vi "rsscope_core_global.vi"() -> ()   [LabVIEW 2014] (continued)
"Access"=2, "Range Table"="", "Read Callback"="rsscope_FormatSearchNameString_ReadCallback.vi", "Write Callback"="rsscope_FormatSearchNameString_WriteCallback.vi", "Supported Models"="", "Instrument Options"="K44", "Flags"=0, "Help"="Specifies the CRC bit pattern, or sets the start value of a pattern range.\n\nAvailable Repeated Capabilities:\nNone\n\nRemote-control command(s):\nSEARch:TRIGger:MPHY:CRC:MIN"}, {"Level"=4, "Class Only"=FALSE, "Identifier"="RSSCOPE_ATTR_SEARCH_MPHY_CRC_MAX", "Descriptive Name"="Search MPHY CRC Max", "Data Type"=2, "Command"="SEAR:TRIG:MPHY:CRC:MAX", "Access"=2, "Range Table"="", "Read Callback"="rsscope_FormatSearchNameString_ReadCallback.vi", "Write Callback"="rsscope_FormatSearchNameString_WriteCallback.vi", "Supported Models"="", "Instrument Options"="K44", "Flags"=0, "Help"="Sets the end value of the CRC range if SEARch:TRIGger:MPHY:CRC:CONDition is set to In Range or Out Of Range.\n\nAvailable Repeated Capabilities:\nNone\n\nRemote-control command(s):\nSEARch:TRIGger:MPHY:CRC:MAX"}, {"Level"=4, "Class Only"=FALSE, "Identifier"="RSSCOPE_ATTR_SEARCH_MPHY_CREQ_PATTERN", "Descriptive Name"="Search MPHY CREQ Pattern", "Data Type"=0, "Command"="SEAR:TRIG:MPHY:CREQ", "Access"=2, "Range Table"="RsScope_rngMPHYREQPattern", "Read Callback"="rsscope_FormatSearchNameInt32_ReadCallback.vi", "Write Callback"="rsscope_FormatSearchNameInt32_WriteCallback.vi", "Supported Models"="", "Instrument Options"="K44", "Flags"=0, "Help"="Specifies the CREQ bit pattern.\n\nAvailable Repeated Capabilities:\nNone\n\nRemote-control command(s):\nSEARch:TRIGger:MPHY:CREQ"}, {"Level"=4, "Class Only"=FALSE, "Identifier"="RSSCOPE_ATTR_SEARCH_MPHY_RREQ_PATTERN", "Descriptive Name"="Search MPHY RREQ Pattern", "Data Type"=0, "Command"="SEAR:TRIG:MPHY:RREQ", "Access"=2, "Range Table"="RsScope_rngMPHYREQPattern", "Read Callback"="rsscope_FormatSearchNameInt32_ReadCallback.vi", "Write Callback"="rsscope_FormatSearchNameInt32_WriteCallback.vi", "Supported Models"="", "Instrument Options"="K44", "Flags"=0, "Help"="Specifies the RREQ bit pattern.\n\nAvailable Repeated Capabilities:\nNone\n\nRemote-control command(s):\nSEARch:TRIGger:MPHY:RREQ"}, {"Level"=4, "Class Only"=FALSE, "Identifier"="RSSCOPE_ATTR_SEARCH_MPHY_CREDIT_CONDITION", "Descriptive Name"="Search MPHY Credit Condition", "Data Type"=0, "Command"="SEAR:TRIG:MPHY:CRED:COND", "Access"=2, "Range Table"="RsScope_rngMPHYWordCondition", "Read Callback"="rsscope_FormatSearchNameInt32_ReadCallback.vi", "Write Callback"="rsscope_FormatSearchNameInt32_WriteCallback.vi", "Supported Models"="", "Instrument Options"="K44", "Flags"=0, "Help"="Sets the condition for Credit. You can define an exact value or a value range.\n\nAvailable Repeated Capabilities:\nNone\n\nRemote-control command(s):\nSEARch:TRIGger:MPHY:CREDit:CONDition"}, {"Level"=4, "Class Only"=FALSE, "Identifier"="RSSCOPE_ATTR_SEARCH_MPHY_CREDIT_MIN", "Descriptive Name"="Search MPHY Credit Min", "Data Type"=2, "Command"="SEAR:TRIG:MPHY:CRED:MIN", "Access"=2, "Range Table"="", "Read Callback"="rsscope_FormatSearchNameString_ReadCallback.vi", "Write Callback"="rsscope_FormatSearchNameString_WriteCallback.vi", "Supported Models"="", "Instrument Options"="K44", "Flags"=0, "Help"="Specifies the Credit bit pattern, or sets the start value of a pattern range.\n\nAvailable Repeated Capabilities:\nNone\n\nRemote-control command(s):\nSEARch:TRIGger:MPHY:CREDit:MIN"}, {"Level"=4, "Class Only"=FALSE, "Identifier"="RSSCOPE_ATTR_SEARCH_MPHY_CREDIT_MAX", "Descriptive Name"="Search MPHY Credit Max", "Data Type"=2, "Command"="SEAR:TRIG:MPHY:CRED:MAX", "Access"=2, "Range Table"="", "Read Callback"="rsscope_FormatSearchNameString_ReadCallback.vi", "Write Callback"="rsscope_FormatSearchNameString_WriteCallback.vi", "Supported Models"="", "Instrument Options"="K44", "Flags"=0, "Help"="Sets the end value of the Credit range if SEARch:TRIGger:MPHY:CREDit:CONDition is set to In Range or Out Of Range.\n\nAvailable Repeated Capabilities:\nNone\n\nRemote-control command(s):\nSEARch:TRIGger:MPHY:CREDit:MAX"}, {"Level"=4, "Class Only"=FALSE, "Identifier"="RSSCOPE_ATTR_SEARCH_MPHY_PACP_BEGIN_CONDITION", "Descriptive Name"="Search MPHY PACP Begin Condition", "Data Type"=0, "Command"="SEAR:TRIG:MPHY:PBEG:COND", "Access"=2, "Range Table"="RsScope_rngMPHYWordCondition", "Read Callback"="rsscope_FormatSearchNameInt32_ReadCallback.vi", "Write Callback"="rsscope_FormatSearchNameInt32_WriteCallback.vi", "Supported Models"="", "Instrument Options"="K44", "Flags"=0, "Help"="Sets the condition for PACP Begin. You can define an exact value or a value range.\n\nAvailable Repeated Capabilities:\nNone\n\nRemote-control command(s):\nSEARch:TRIGger:MPHY:PBEGin:CONDition"}, {"Level"=4, "Class Only"=FALSE, "Identifier"="RSSCOPE_ATTR_SEARCH_MPHY_PACP_BEGIN_MIN", "Descriptive Name"="Search MPHY PACP Begin Min", "Data Type"=2, "Command"="SEAR:TRIG:MPHY:PBEG:MIN", "Access"=2, "Range Table"="", "Read Callback"="rsscope_FormatSearchNameString_ReadCallback.vi", "Write Callback"="rsscope_FormatSearchNameString_WriteCallback.vi", "Supported Models"="", "Instrument Options"="K44", "Flags"=0, "Help"="Specifies the PACP Begin bit pattern, or sets the start value of a pattern range.\n\nAvailable Repeated Capabilities:\nNone\n\nRemote-control command(s):\nSEARch:TRIGger:MPHY:PBEGin:MIN"}, {"Level"=4, "Class Only"=FALSE, "Identifier"="RSSCOPE_ATTR_SEARCH_MPHY_PACP_BEGIN_MAX", "Descriptive Name"="Search MPHY PACP Begin Max", "Data Type"=2, "Command"="SEAR:TRIG:MPHY:PBEG:MAX", "Access"=2, "Range Table"="", "Read Callback"="rsscope_FormatSearchNameString_ReadCallback.vi", "Write Callback"="rsscope_FormatSearchNameString_WriteCallback.vi", "Supported Models"="", "Instrument Options"="K44", "Flags"=0, "Help"="Sets the end value of the PACP Begin range if SEARch:TRIGger:MPHY:PBEGin:CONDition is set to In Range or Out Of Range.\n\nAvailable Repeated Capabilities:\nNone\n\nRemote-control command(s):\nSEARch:TRIGger:MPHY:PBEGin:MAX"}, {"Level"=4, "Class Only"=FALSE, "Identifier"="RSSCOPE_ATTR_SEARCH_MPHY_PACP_ID_CONDITION", "Descriptive Name"="Search MPHY PACP ID Condition", "Data Type"=0, "Command"="SEAR:TRIG:MPHY:PFID:COND", "Access"=2, "Range Table"="RsScope_rngMPHYWordCondition", "Read Callback"="rsscope_FormatSearchNameInt32_ReadCallback.vi", "Write Callback"="rsscope_FormatSearchNameInt32_WriteCallback.vi", "Supported Models"="", "Instrument Options"="K44", "Flags"=0, "Help"="Sets the condition for PACP Function ID. You can define an exact value or a value range.\n\nAvailable Repeated Capabilities:\nNone\n\nRemote-control command(s):\nSEARch:TRIGger:MPHY:PFID:CONDition"}, {"Level"=4, "Class Only"=FALSE, "Identifier"="RSSCOPE_ATTR_SEARCH_MPHY_PACP_ID_MIN", "Descriptive Name"="Search MPHY PACP ID Min", "Data Type"=2, "Command"="SEAR:TRIG:MPHY:PFID:MIN", "Access"=2, "Range Table"="", "Read Callback"="rsscope_FormatSearchNameString_ReadCallback.vi", "Write Callback"="rsscope_FormatSearchNameString_WriteCallback.vi", "Supported Models"="", "Instrument Options"="K44", "Flags"=0, "Help"="Specifies the PACP Function ID bit pattern, or sets the start value of a pattern range.\n\nAvailable Repeated Capabilities:\nNone\n\nRemote-control command(s):\nSEARch:TRIGger:MPHY:PFID:MIN"}, {"Level"=4, "Class Only"=FALSE, "Identifier"="RSSCOPE_ATTR_SEARCH_MPHY_PACP_ID_MAX", "Descriptive Name"="Search MPHY PACP ID Max", "Data Type"=2, "Command"="SEAR:TRIG:MPHY:PFID:MAX", "Access"=2, "Range Table"="", "Read Callback"="rsscope_FormatSearchNameString_ReadCallback.vi", "Write Callback"="rsscope_FormatSearchNameString_WriteCallback.vi", "Supported Models"="", "Instrument Options"="K44", "Flags"=0, "Help"="Sets the end value of the PACP Function ID range if SEARch:TRIGger:MPHY:PFID:CONDition is set to In Range or Out Of Range.\n\nAvailable Repeated Capabilities:\nNone\n\nRemote-control command(s):\nSEARch:TRIGger:MPHY:PFID:MAX"}, {"Level"=4, "Class Only"=FALSE, "Identifier"="RSSCOPE_ATTR_SEARCH_MPHY_LCC_ERROR", "Descriptive Name"="Search MPHY LCC Error", "Data Type"=3, "Command"="SEAR:TRIG:MPHY:ERR:LCMD", "Access"=2, "Range Table"="", "Read Callback"="rsscope_FormatSearchNameBoolean_ReadCallback.vi", "Write Callback"="rsscope_FormatSearchNameBoolean_WriteCallback.vi", "Supported Models"="", "Instrument Options"="K44", "Flags"=0, "Help"="Enables or disables search for LCC error.\n\nAvailable Repeated Capabilities:\nNone\n\nRemote-control command(s):\nSEARch:TRIGger:MPHY:ERRor:LCMD"}, {"Level"=4, "Class Only"=FALSE, "Identifier"="RSSCOPE_ATTR_SEARCH_MPHY_ERROR_LENGTH", "Descriptive Name"="Search MPHY Error Length", "Data Type"=3, "Command"="SEAR:TRIG:MPHY:ERR:LENG", "Access"=2, "Range Table"="", "Read Callback"="rsscope_FormatSearchNameBoolean_ReadCallback.vi", "Write Callback"="rsscope_FormatSearchNameBoolean_WriteCallback.vi", "Supported Models"="", "Instrument Options"="K44", "Flags"=0, "Help"="Enables or disables search for length error.\n\nAvailable Repeated Capabilities:\nNone\n\nRemote-control command(s):\nSEARch:TRIGger:MPHY:ERRor:LENGth"}, {"Level"=4, "Class Only"=FALSE, "Identifier"="RSSCOPE_ATTR_SEARCH_MPHY_ERROR_RESERVED", "Descriptive Name"="Search MPHY Error Reserved", "Data Type"=3, "Command"="SEAR:TRIG:MPHY:ERR:RES", "Access"=2, "Range Table"="", "Read Callback"="rsscope_FormatSearchNameBoolean_ReadCallback.vi", "Write Callback"="rsscope_FormatSearchNameBoolean_WriteCallback.vi", "Supported Models"="", "Instrument Options"="K44", "Flags"=0, "Help"="Enables or disables search for reserved bit error.\n\nAvailable Repeated Capabilities:\nNone\n\nRemote-control command(s):\nSEARch:TRIGger:MPHY:ERRor:REServed"}, {"Level"=4, "Class Only"=FALSE, "Identifier"="RSSCOPE_ATTR_SEARCH_MPHY_ERROR_SYMBOL", "Descriptive Name"="Search MPHY Error Symbol", "Data Type"=3, "Command"="SEAR:TRIG:MPHY:ERR:SYMB", "Access"=2, "Range Table"="", "Read Callback"="rsscope_FormatSearchNameBoolean_ReadCallback.vi", "Write Callback"="rsscope_FormatSearchNameBoolean_WriteCallback.vi", "Supported Models"="", "Instrument Options"="K44", "Flags"=0, "Help"="Enables or disables search for 8b10b symbol error.\n\nAvailable Repeated Capabilities:\nNone\n\nRemote-control command(s):\nSEARch:TRIGger:MPHY:ERRor:SYMBol"}, {"Level"=4, "Class Only"=FALSE, "Identifier"="RSSCOPE_ATTR_SEARCH_MPHY_ERROR_UNIDENTIFIED_UNIPRO_FRAME", "Descriptive Name"="Search MPHY Error Unidentified UniPro Frame", "Data Type"=3, "Command"="SEAR:TRIG:MPHY:ERR:UNKN", "Access"=2, "Range Table"="", "Read Callback"="rsscope_FormatSearchNameBoolean_ReadCallback.vi", "Write Callback"="rsscope_FormatSearchNameBoolean_WriteCallback.vi", "Supported Models"="", "Instrument Options"="K44", "Flags"=0, "Help"="Enables or disables search for unidentified UniPro frame error.\n\nAvailable Repeated Capabilities:\nNone\n\nRemote-control command(s):\nSEARch:TRIGger:MPHY:ERRor:UNKNown"}, {"Level"=4, "Class Only"=TRUE, "Identifier"="", "Descriptive Name"="SSIC", "Data Type"=0, "Command"="", "Access"=0, "Range Table"="", "Read Callback"="", "Write Callback"="", "Supported Models"="", "Instrument Options"="", "Flags"=0, "Help"="Search Settings USB SSIC"}, {"Level"=4, "Class Only"=TRUE, "Identifier"="", "Descriptive Name"="Results", "Data Type"=0, "Command"="", "Access"=0, "Range Table"="", "Read Callback"="", "Write Callback"="", "Supported Models"="", "Instrument Options"="", "Flags"=0, "Help"="Returns the M-PHY search results."}, {"Level"=3, "Class Only"=TRUE, "Identifier"="", "Descriptive Name"="CXPI", "Data Type"=0, "Command"="", "Access"=0, "Range Table"="", "Read Callback"="", "Write Callback"="", "Supported Models"="", "Instrument Options"="", "Flags"=0, "Help"="Configures CXPI search."}, {"Level"=4, "Class Only"=FALSE, "Identifier"="RSSCOPE_ATTR_CXPI_SEARCH_TYPE", "Descriptive Name"="CXPI Search Type", "Data Type"=0, "Command"="SEAR:TRIG:CXPI:TYPE", "Access"=2, "Range Table"="RsScope_rngCXPITriggerType", "Read Callback"="rsscope_FormatSearchNameInt32_ReadCallback.vi", "Write Callback"="rsscope_FormatSearchNameInt32_WriteCallback.vi", "Supported Models"="", "Instrument Options"="K76", "Flags"=0, "Help"="Selects the trigger type for the CXPI analysis.\n\nAvailable Repeated Capabilities:\nNone\n\nRemote-control command(s):\nSEARch:TRIGger:CXPI:TYPE"}, {"Level"=4, "Class Only"=FALSE, "Identifier"="RSSCOPE_ATTR_CXPI_SEARCH_NM", "Descriptive Name"="CXPI Search NM", "Data Type"=2, "Command"="SEAR:TRIG:CXPI:NM", "Access"=2, "Range Table"="", "Read Callback"="rsscope_FormatSearchNameString_ReadCallback.vi", "Write Callback"="rsscope_FormatSearchNameString_WriteCallback.vi", "Supported Models"="", "Instrument Options"="K76", "Flags"=0, "Help"="Sets the value of the network management (NM) field.\n\nAvailable Repeated Capabilities:\nNone\n\nRemote-control command(s):\nSEARch:TRIGger:CXPI:NM"}, {"Level"=4, "Class Only"=FALSE, "Identifier"="RSSCOPE_ATTR_CXPI_SEARCH_CT", "Descriptive Name"="CXPI Search CT", "Data Type"=2, "Command"="SEAR:TRIG:CXPI:CT", "Access"=2, "Range Table"="", "Read Callback"="rsscope_FormatSearchNameString_ReadCallback.vi", "Write Callback"="rsscope_FormatSearchNameString_WriteCallback.vi", "Supported Models"="", "Instrument Options"="K76", "Flags"=0, "Help"="Sets the value of the counter (CT), 2 bits indicating the continuity of the frame.\n\nAvailable Repeated Capabilities:\nNone\n\nRemote-control command(s):\nSEARch:TRIGger:CXPI:CT"}, {"Level"=4, "Class Only"=TRUE, "Identifier"="", "Descriptive Name"="Frame ID", "Data Type"=0, "Command"="", "Access"=0, "Range Table"="", "Read Callback"="", "Write Callback"="", "Supported Models"="", "Instrument Options"="", "Flags"=0, "Help"="The frame identifier is a 7-bit field. Its setup consists of the condition and one or two frame patterns."}, {"Level"=5, "Class Only"=FALSE, "Identifier"="RSSCOPE_ATTR_CXPI_SEARCH_FRAME_ID_CONDITION", "Descriptive Name"="CXPI Search Frame ID Condition", "Data Type"=0, "Command"="SEAR:TRIG:CXPI:FID:COND", "Access"=2, "Range Table"="rsscope_rngProtocolTriggerCondition", "Read Callback"="rsscope_FormatSearchNameInt32_ReadCallback.vi", "Write Callback"="rsscope_FormatSearchNameInt32_WriteCallback.vi", "Supported Models"="", "Instrument Options"="K76", "Flags"=0, "Help"="Set the condition for the frame ID. You can define an exact value or a value range.\n\nAvailable Repeated Capabilities:\nNone\n\nRemote-control command(s):\nSEARch:TRIGger:CXPI:FID:CONDition"}, {"Level"=5, "Class Only"=FALSE, "Identifier"="RSSCOPE_ATTR_CXPI_SEARCH_FRAME_ID_MIN", "Descriptive Name"="CXPI Search Frame ID Min", "Data Type"=2, "Command"="SEAR:TRIG:CXPI:FID:MIN", "Access"=2, "Range Table"="", "Read Callback"="rsscope_FormatSearchNameString_ReadCallback.vi", "Write Callback"="rsscope_FormatSearchNameString_WriteCallback.vi", "Supported Models"="", "Instrument Options"="K76", "Flags"=0, "Help"="Specifies a frame ID pattern, or sets the start value of a pattern range.\n\nValid Values:\nBinary pattern string consisting of 1; 0; or X (any bit).\n\nAvailable Repeated Capabilities:\nNone\n\nRemote-control command(s):\nSEARch:TRIGger:CXPI:FID:MIN"}, {"Level"=5, "Class Only"=FALSE, "Identifier"="RSSCOPE_ATTR_CXPI_SEARCH_FRAME_ID_MAX", "Descriptive Name"="CXPI Search Frame ID Max", "Data Type"=2, "Command"="SEAR:TRIG:CXPI:FID:MAX", "Access"=2, "Range Table"="", "Read Callback"="rsscope_FormatSearchNameString_ReadCallback.vi", "Write Callback"="rsscope_FormatSearchNameString_WriteCallback.vi", "Supported Models"="", "Instrument Options"="K76", "Flags"=0, "Help"="Sets the end value of a frame ID range for condition In Range or Out of Range. \n\nValid Values:\nBinary pattern string consisting of 1; 0; or X (any bit).\n\nAvailable Repeated Capabilities:\nNone\n\nRemote-control command(s):\nSEARch:TRIGger:CXPI:FID:MAX"}, {"Level"=4, "Class Only"=TRUE, "Identifier"="", "Descriptive Name"="DLC", "Data Type"=0, "Command"="", "Access"=0, "Range Table"="", "Read Callback"="", "Write Callback"="", "Supported Models"="", "Instrument Options"="", "Flags"=0, "Help"="Sets the data length code, which indicates the length of the data byte."}, {"Level"=5, "Class Only"=FALSE, "Identifier"="RSSCOPE_ATTR_CXPI_SEARCH_DLC_CONDITION", "Descriptive Name"="CXPI Search DLC Condition", "Data Type"=0, "Command"="SEAR:TRIG:CXPI:DLC:COND", "Access"=2, "Range Table"="rsscope_rngProtocolTriggerCondition", "Read Callback"="rsscope_FormatSearchNameInt32_ReadCallback.vi", "Write Callback"="rsscope_FormatSearchNameInt32_WriteCallback.vi", "Supported Models"="", "Instrument Options"="K76", "Flags"=0, "Help"="Set the condition for the DLC. You can define an exact value or a value range.\n\nAvailable Repeated Capabilities:\nNone\n\nRemote-control command(s):\nSEARch:TRIGger:CXPI:DLC:CONDition"}, {"Level"=5, "Class Only"=FALSE, "Identifier"="RSSCOPE_ATTR_CXPI_SEARCH_DLC_MIN", "Descriptive Name"="CXPI Search DLC Min", "Data Type"=2, "Command"="SEAR:TRIG:CXPI:DLC:MIN", "Access"=2, "Range Table"="", "Read Callback"="rsscope_FormatSearchNameString_ReadCallback.vi", "Write Callback"="rsscope_FormatSearchNameString_WriteCallback.vi", "Supported Models"="", "Instrument Options"="K76", "Flags"=0, "Help"="Specifies a DLC pattern, or sets the start value of a pattern range.\n\nValid Values:\nBinary pattern string consisting of 1; 0; or X (any bit).\n\nAvailable Repeated Capabilities:\nNone\n\nRemote-control command(s):\nSEARch:TRIGger:CXPI:DLC:MIN"}, {"Level"=5, "Class Only"=FALSE, "Identifier"="RSSCOPE_ATTR_CXPI_SEARCH_DLC_MAX", "Descriptive Name"="CXPI Search DLC Max", "Data Type"=2, "Command"="SEAR:TRIG:CXPI:DLC:MAX", "Access"=2, "Range Table"="", "Read Callback"="rsscope_FormatSearchNameString_ReadCallback.vi", "Write Callback"="rsscope_FormatSearchNameString_WriteCallback.vi", "Supported Models"="", "Instrument Options"="K76", "Flags"=0, "Help"="Sets the end value of a data type range for condition In Range or Out of Range. \n\nValid Values:\nBinary pattern string consisting of 1; 0; or X (any bit).\n\nAvailable Repeated Capabilities:\nNone\n\nRemote-control command(s):\nSEARch:TRIGger:CXPI:DLC:MAX"}, {"Level"=4, "Class Only"=TRUE, "Identifier"="", "Descriptive Name"="DLC Extend", "Data Type"=0, "Command"="", "Access"=0, "Range Table"="", "Read Callback"="", "Write Callback"="", "Supported Models"="", "Instrument Options"="", "Flags"=0, "Help"="Sets the extension data length code, which indicates the length of the data byte of a long frame."}, {"Level"=5, "Class Only"=FALSE, "Identifier"="RSSCOPE_ATTR_CXPI_SEARCH_DLC_EXTEND_CONDITION", "Descriptive Name"="CXPI Search DLC Extend Condition", "Data Type"=0, "Command"="SEAR:TRIG:CXPI:DEXT:COND", "Access"=2, "Range Table"="rsscope_rngProtocolTriggerCondition", "Read Callback"="rsscope_FormatSearchNameInt32_ReadCallback.vi", "Write Callback"="rsscope_FormatSearchNameInt32_WriteCallback.vi", "Supported Models"="", "Instrument Options"="K76", "Flags"=0, "Help"="Set the condition for the DLC extend value. You can define an exact value or a value range.\n\nAvailable Repeated Capabilities:\nNone\n\nRemote-control command(s):\nSEARch:TRIGger:CXPI:DEXTension:CONDition"}, {"Level"=5, "Class Only"=FALSE, "Identifier"="RSSCOPE_ATTR_CXPI_SEARCH_DLC_EXTEND_MIN", "Descriptive Name"="CXPI Search DLC Extend Min", "Data Type"=2, "Command"="SEAR:TRIG:CXPI:DEXT:MIN", "Access"=2, "Range Table"="", "Read Callback"="rsscope_FormatSearchNameString_ReadCallback.vi", "Write Callback"="rsscope_FormatSearchNameString_WriteCallback.vi", "Supported Models"="", "Instrument Options"="K76", "Flags"=0, "Help"="Specifies a data extension bit pattern, or sets the start value of a pattern range.\n\nValid Values:\nBinary pattern string consisting of 1; 0; or X (any bit).\n\nAvailable Repeated Capabilities:\nNone\n\nRemote-control command(s):\nSEARch:TRIGger:CXPI:DEXTension:MIN"}, {"Level"=5, "Class Only"=FALSE, "Identifier"="RSSCOPE_ATTR_CXPI_SEARCH_DLC_EXTEND_MAX", "Descriptive Name"="CXPI Search DLC Extend Max", "Data Type"=2, "Command"="SEAR:TRIG:CXPI:DEXT:MAX", "Access"=2, "Range Table"="", "Read Callback"="rsscope_FormatSearchNameString_ReadCallback.vi", "Write Callback"="rsscope_FormatSearchNameString_WriteCallback.vi", "Supported Models"="", "Instrument Options"="K76", "Flags"=0, "Help"="Sets the end value of a DLC extend range for condition In Range or Out of Range. \n\nValid Values:\nBinary pattern string consisting of 1; 0; or X (any bit).\n\nAvailable Repeated Capabilities:\nNone\n\nRemote-control command(s):\nSEARch:TRIGger:CXPI:DEXTension:MAX"}, {"Level"=4, "Class Only"=TRUE, "Identifier"="", "Descriptive Name"="Data", "Data Type"=0, "Command"="", "Access"=0, "Range Table"="", "Read Callback"="", "Write Callback"="", "Supported Models"="", "Instrument Options"="", "Flags"=0, "Help"="The data setup consists of the condition and one or two identifier pattern."}, {"Level"=5, "Class Only"=FALSE, "Identifier"="RSSCOPE_ATTR_CXPI_SEARCH_DATA_CONDITION", "Descriptive Name"="CXPI Search Data Condition", "Data Type"=0, "Command"="SEAR:TRIG:CXPI:DATA:DCON", "Access"=2, "Range Table"="rsscope_rngCXPIDataCondition", "Read Callback"="rsscope_FormatSearchNameInt32_ReadCallback.vi", "Write Callback"="rsscope_FormatSearchNameInt32_WriteCallback.vi", "Supported Models"="", "Instrument Options"="K76", "Flags"=0, "Help"="Sets the condition for the data pattern. You can define no value, an exact value or a value range.\n\nAvailable Repeated Capabilities:\nNone\n\nRemote-control command(s):\nSEARch:TRIGger:CXPI:DATA:DCONdition"}, {"Level"=5, "Class Only"=FALSE, "Identifier"="RSSCOPE_ATTR_CXPI_SEARCH_DATA_MIN", "Descriptive Name"="CXPI Search Data Min", "Data Type"=2, "Command"="SEAR:TRIG:CXPI:DATA:DMIN", "Access"=2, "Range Table"="", "Read Callback"="rsscope_FormatSearchNameString_ReadCallback.vi", "Write Callback"="rsscope_FormatSearchNameString_WriteCallback.vi", "Supported Models"="", "Instrument Options"="K76", "Flags"=0, "Help"="Specifies a data bit pattern, or sets the start value of a pattern range.\n\nValid Values:\nBinary pattern string consisting of 1; 0; or X (any bit).\n\nAvailable Repeated Capabilities:\nNone\n\nRemote-control command(s):\nSEARch:TRIGger:CXPI:DATA:DMIN"}, {"Level"=5, "Class Only"=FALSE, "Identifier"="RSSCOPE_ATTR_CXPI_SEARCH_DATA_MAX", "Descriptive Name"="CXPI Search Data Max", "Data Type"=2, "Command"="SEAR:TRIG:CXPI:DATA:DMAX", "Access"=2, "Range Table"="", "Read Callback"="rsscope_FormatSearchNameString_ReadCallback.vi", "Write Callback"="rsscope_FormatSearchNameString_WriteCallback.vi", "Supported Models"="", "Instrument Options"="K76", "Flags"=0, "Help"="Sets the end value of a data type range for condition In Range or Out of Range. \n\nValid Values:\nBinary pattern string consisting of 1; 0; or X (any bit).\n\nAvailable Repeated Capabilities:\nNone\n\nRemote-control command(s):\nSEARch:TRIGger:CXPI:DATA:DMAX"}, {"Level"=4, "Class Only"=TRUE, "Identifier"="", "Descriptive Name"="Index", "Data Type"=0, "Command"="", "Access"=0, "Range Table"="", "Read Callback"="", "Write Callback"="", "Supported Models"="", "Instrument Options"="", "Flags"=0, "Help"="The data index setup consists of the condition and one or two index patterns."}, {"Level"=5, "Class Only"=FALSE, "Identifier"="RSSCOPE_ATTR_CXPI_SEARCH_INDEX_CONDITION", "Descriptive Name"="CXPI Search Index Condition", "Data Type"=0, "Command"="SEAR:TRIG:CXPI:DATA:ICON", "Access"=2, "Range Table"="rsscope_rngProtocolTriggerCondition", "Read Callback"="rsscope_FormatSearchNameInt32_ReadCallback.vi", "Write Callback"="rsscope_FormatSearchNameInt32_WriteCallback.vi", "Supported Models"="", "Instrument Options"="K76", "Flags"=0, "Help"="Set the condition for the data index value. You can define an exact value or a value range.\n\nAvailable Repeated Capabilities:\nNone\n\nRemote-control command(s):\nSEARch:TRIGger:CXPI:DATA:ICONdition"}, {"Level"=5, "Class Only"=FALSE, "Identifier"="RSSCOPE_ATTR_CXPI_SEARCH_INDEX_MIN", "Descriptive Name"="CXPI Search Index Min", "Data Type"=0, "Command"="SEAR:TRIG:CXPI:DATA:IMIN", "Access"=2, "Range Table"="", "Read Callback"="rsscope_FormatSearchNameInt32_ReadCallback.vi", "Write Callback"="rsscope_FormatSearchNameInt32_WriteCallback.vi", "Supported Models"="", "Instrument Options"="K76", "Flags"=0, "Help"="Specifies a data index bit pattern, or sets the start value of a pattern range.\n\nAvailable Repeated Capabilities:\nNone\n\nRemote-control command(s):\nSEARch:TRIGger:CXPI:DATA:IMIN"}, {"Level"=5, "Class Only"=FALSE, "Identifier"="RSSCOPE_ATTR_CXPI_SEARCH_INDEX_MAX", "Descriptive Name"="CXPI Search Index Max", "Data Type"=0, "Command"="SEAR:TRIG:CXPI:DATA:IMAX", "Access"=2, "Range Table"="", "Read Callback"="rsscope_FormatSearchNameInt32_ReadCallback.vi", "Write Callback"="rsscope_FormatSearchNameInt32_WriteCallback.vi", "Supported Models"="", "Instrument Options"="K76", "Flags"=0, "Help"="Sets the end value of a data index range for condition In Range or Out of Range.\n\nAvailable Repeated Capabilities:\nNone\n\nRemote-control command(s):\nSEARch:TRIGger:CXPI:DATA:IMAX"}, {"Level"=4, "Class Only"=TRUE, "Identifier"="", "Descriptive Name"="Error", "Data Type"=0, "Command"="", "Access"=0, "Range Table"="", "Read Callback"="", "Write Callback"="", "Supported Models"="", "Instrument Options"="", "Flags"=0, "Help"="Trigger on selected error types."}, {"Level"=5, "Class Only"=FALSE, "Identifier"="RSSCOPE_ATTR_CXPI_SEARCH_ERROR_CRC", "Descriptive Name"="CXPI Search Error CRC", "Data Type"=3, "Command"="SEAR:TRIG:CXPI:ERR:CRC", "Access"=2, "Range Table"="", "Read Callback"="rsscope_FormatSearchNameBoolean_ReadCallback.vi", "Write Callback"="rsscope_FormatSearchNameBoolean_WriteCallback.vi", "Supported Models"="", "Instrument Options"="K76", "Flags"=0, "Help"="Searches for a cyclic redundancy check error.\n\nAvailable Repeated Capabilities:\nNone\n\nRemote-control command(s):\nSEARch:TRIGger:CXPI:ERRor:CRC"}, {"Level"=5, "Class Only"=FALSE, "Identifier"="RSSCOPE_ATTR_CXPI_SEARCH_ERROR_DLC", "Descriptive Name"="CXPI Search Error DLC", "Data Type"=3, "Command"="SEAR:TRIG:CXPI:ERR:DLC", "Access"=2, "Range Table"="", "Read Callback"="rsscope_FormatSearchNameBoolean_ReadCallback.vi", "Write Callback"="rsscope_FormatSearchNameBoolean_WriteCallback.vi", "Supported Models"="", "Instrument Options"="K76", "Flags"=0, "Help"="Searches for a data length code (DLC) error.\n\nAvailable Repeated Capabilities:\nNone\n\nRemote-control command(s):\nSEARch:TRIGger:CXPI:ERRor:DLC"}, {"Level"=5, "Class Only"=FALSE, "Identifier"="RSSCOPE_ATTR_CXPI_SEARCH_ERROR_IBS", "Descriptive Name"="CXPI Search Error IBS", "Data Type"=3, "Command"="SEAR:TRIG:CXPI:ERR:IBS", "Access"=2, "Range Table"="", "Read Callback"="rsscope_FormatSearchNameBoolean_ReadCallback.vi", "Write Callback"="rsscope_FormatSearchNameBoolean_WriteCallback.vi", "Supported Models"="", "Instrument Options"="K76", "Flags"=0, "Help"="Searches for an inter-byte-space (IBS) error.\n\nAvailable Repeated Capabilities:\nNone\n\nRemote-control command(s):\nSEARch:TRIGger:CXPI:ERRor:IBS"}, {"Level"=5, "Class Only"=FALSE, "Identifier"="RSSCOPE_ATTR_CXPI_SEARCH_ERROR_IFS", "Descriptive Name"="CXPI Search Error IFS", "Data Type"=3, "Command"="SEAR:TRIG:CXPI:ERR:IFS", "Access"=2, "Range Table"="", "Read Callback"="rsscope_FormatSearchNameBoolean_ReadCallback.vi", "Write Callback"="rsscope_FormatSearchNameBoolean_WriteCallback.vi", "Supported Models"="", "Instrument Options"="K76", "Flags"=0, "Help"="Searches for an inter-frame-space (IFS) error.\n\nAvailable Repeated Capabilities:\nNone\n\nRemote-control command(s):\nSEARch:TRIGger:CXPI:ERRor:IFS"}, {"Level"=5, "Class Only"=FALSE, "Identifier"="RSSCOPE_ATTR_CXPI_SEARCH_ERROR_LENGTH", "Descriptive Name"="CXPI Search Error Length", "Data Type"=3, "Command"="SEAR:TRIG:CXPI:ERR:LENG", "Access"=2, "Range Table"="", "Read Callback"="rsscope_FormatSearchNameBoolean_ReadCallback.vi", "Write Callback"="rsscope_FormatSearchNameBoolean_WriteCallback.vi", "Supported Models"="", "Instrument Options"="K76", "Flags"=0, "Help"="Searches for a length error.\n\nAvailable Repeated Capabilities:\nNone\n\nRemote-control command(s):\nSEARch:TRIGger:CXPI:ERRor:LENGth"}, {"Level"=5, "Class Only"=FALSE, "Identifier"="RSSCOPE_ATTR_CXPI_SEARCH_ERROR_PARITY", "Descriptive Name"="CXPI Search Error Parity", "Data Type"=3, "Command"="SEAR:TRIG:CXPI:ERR:PAR", "Access"=2, "Range Table"="", "Read Callback"="rsscope_FormatSearchNameBoolean_ReadCallback.vi", "Write Callback"="rsscope_FormatSearchNameBoolean_WriteCallback.vi", "Supported Models"="", "Instrument Options"="K76", "Flags"=0, "Help"="Searches for a parity error indicating a transmission error.\n\nAvailable Repeated Capabilities:\nNone\n\nRemote-control command(s):\nSEARch:TRIGger:CXPI:ERRor:PARity"}, {"Level"=5, "Class Only"=FALSE, "Identifier"="RSSCOPE_ATTR_CXPI_SEARCH_ERROR_UART", "Descriptive Name"="CXPI Search Error UART", "Data Type"=3, "Command"="SEAR:TRIG:CXPI:ERR:UART", "Access"=2, "Range Table"="", "Read Callback"="rsscope_FormatSearchNameBoolean_ReadCallback.vi", "Write Callback"="rsscope_FormatSearchNameBoolean_WriteCallback.vi", "Supported Models"="", "Instrument Options"="K76", "Flags"=0, "Help"="Searches for an UART error.\n\nAvailable Repeated Capabilities:\nNone\n\nRemote-control command(s):\nSEARch:TRIGger:CXPI:ERRor:UART"}, {"Level"=4, "Class Only"=TRUE, "Identifier"="", "Descriptive Name"="Results", "Data Type"=0, "Command"="", "Access"=0, "Range Table"="", "Read Callback"="", "Write Callback"="", "Supported Models"="", "Instrument Options"="", "Flags"=0, "Help"="Searches the CXPI decoding results."}, {"Level"=5, "Class Only"=FALSE, "Identifier"="RSSCOPE_ATTR_SEARCH_CXPI_FRAME_COUNT", "Descriptive Name"="Search CXPI Frame Count", "Data Type"=0, "Command"="SEAR:RES:CXPI:FCO?", "Access"=0, "Range Table"="", "Read Callback"="rsscope_FormatSearchNameInt32_ReadCallback.vi", "Write Callback"="", "Supported Models"="", "Instrument Options"="K76", "Flags"=0, "Help"="Returns the number of frames in the acquisition.\n\nAvailable Repeated Capabilities:\nNone\n\nRemote-control command(s):\nSEARch:RESult:CXPI:FCOunt?"}, {"Level"=3, "Class Only"=TRUE, "Identifier"="", "Descriptive Name"="PCIe", "Data Type"=0, "Command"="", "Access"=0, "Range Table"="", "Read Callback"="", "Write Callback"="", "Supported Models"="", "Instrument Options"="", "Flags"=0, "Help"="Configures PCIe search."}, {"Level"=4, "Class Only"=FALSE, "Identifier"="RSSCOPE_ATTR_PCIE_SEARCH_TYPE", "Descriptive Name"="PCIe Search Type", "Data Type"=0, "Command"="SEAR:TRIG:PCIE:TYPE", "Access"=2, "Range Table"="RsScope_rngPCIeTriggerType", "Read Callback"="rsscope_FormatSearchNameInt32_ReadCallback.vi", "Write Callback"="rsscope_FormatSearchNameInt32_WriteCallback.vi", "Supported Models"="RTO|RTP", "Instrument Options"="K72", "Flags"=0, "Help"="Sets the trigger type for the PCI express analysis.\n\nAvailable Repeated Capabilities:\nNone\n\nRemote-control command(s):\nSEARch:TRIGger:PCIE:TYPE"}, {"Level"=4, "Class Only"=FALSE, "Identifier"="RSSCOPE_ATTR_PCIE_PACKET_COUNT", "Descriptive Name"="PCIe Packet Count", "Data Type"=0, "Command"="SEAR:RES:PCIE:PCO?", "Access"=0, "Range Table"="", "Read Callback"="rsscope_FormatSearchNameInt32_ReadCallback.vi", "Write Callback"="", "Supported Models"="", "Instrument Options"="", "Flags"=0, "Help"="Returns the packet count for the selected serial bus, i.e. the number of packets in the present acquisition.\n\nAvailable Repeated Capabilities:\nNone\n\nRemote-control command(s):\nSEARch:RESult:PCIE:PCOunt?"}, {"Level"=4, "Class Only"=TRUE, "Identifier"="", "Descriptive Name"="TLP", "Data Type"=0, "Command"="", "Access"=0, "Range Table"="", "Read Callback"="", "Write Callback"="", "Supported Models"="", "Instrument Options"="", "Flags"=0, "Help"="Search on a transaction type."}, {"Level"=5, "Class Only"=FALSE, "Identifier"="RSSCOPE_ATTR_PCIE_SEARCH_TLP", "Descriptive Name"="PCIe Search TLP", "Data Type"=0, "Command"="SEAR:TRIG:PCIE:TLP:TYPE", "Access"=2, "Range Table"="RsScope_rngPCIeTLP", "Read Callback"="rsscope_FormatSearchNameInt32_ReadCallback.vi", "Write Callback"="rsscope_FormatSearchNameInt32_WriteCallback.vi", "Supported Models"="RTO|RTP", "Instrument Options"="K72", "Flags"=0, "Help"="Sets the transaction type to be searched for in the transaction layer type.\n\nAvailable Repeated Capabilities:\nNone\n\nRemote-control command(s):\nSEARch:TRIGger:PCIE:TLP:TYPE"}, {"Level"=5, "Class Only"=FALSE, "Identifier"="RSSCOPE_ATTR_PCIE_SEARCH_TLP_SEQUENCE_NUMBER", "Descriptive Name"="PCIe Search TLP Sequence Number", "Data Type"=2, "Command"="SEAR:TRIG:PCIE:TLP:SNUM", "Access"=2, "Range Table"="", "Read Callback"="rsscope_FormatSearchNameString_ReadCallback.vi", "Write Callback"="rsscope_FormatSearchNameString_WriteCallback.vi", "Supported Models"="RTO|RTP", "Instrument Options"="K72", "Flags"=0, "Help"="Sets the sequence numbe to be searched for in the transaction layer type.\n\nAvailable Repeated Capabilities:\nNone\n\nRemote-control command(s):\nSEARch:TRIGger:PCIE:TLP:SNUM"}, {"Level"=5, "Class Only"=FALSE, "Identifier"="RSSCOPE_ATTR_PCIE_SEARCH_TLP_TC", "Descriptive Name"="PCIe Search TLP TC", "Data Type"=0, "Command"="SEAR:TRIG:PCIE:TLP:TCHN", "Access"=2, "Range Table"="RsScope_rngPCIeTLPTC", "Read Callback"="rsscope_FormatSearchNameInt32_ReadCallback.vi", "Write Callback"="rsscope_FormatSearchNameInt32_WriteCallback.vi", "Supported Models"="RTO|RTP", "Instrument Options"="K72", "Flags"=0, "Help"="Sets the traffic class to be searched for in the transaction layer type.\n\nAvailable Repeated Capabilities:\nNone\n\nRemote-control command(s):\nSEARch:TRIGger:PCIE:TLP:TCHN"}, {"Level"=5, "Class Only"=FALSE, "Identifier"="RSSCOPE_ATTR_PCIE_SEARCH_TLP_ORDERING", "Descriptive Name"="PCIe Search TLP Ordering", "Data Type"=0, "Command"="SEAR:TRIG:PCIE:TLP:ORDE", "Access"=2, "Range Table"="RsScope_rngPCIeTLPOrdering", "Read Callback"="rsscope_FormatSearchNameInt32_ReadCallback.vi", "Write Callback"="rsscope_FormatSearchNameInt32_WriteCallback.vi", "Supported Models"="RTO|RTP", "Instrument Options"="K72", "Flags"=0, "Help"="Sets the ordering type to be searched for in the transaction layer type.\n\nAvailable Repeated Capabilities:\nNone\n\nRemote-control command(s):\nSEARch:TRIGger:PCIE:TLP:ORDE"}, {"Level"=5, "Class Only"=FALSE, "Identifier"="RSSCOPE_ATTR_PCIE_SEARCH_TLP_SNOOP", "Descriptive Name"="PCIe Search TLP Snoop", "Data Type"=0, "Command"="SEAR:TRIG:PCIE:TLP:SNOO", "Access"=2, "Range Table"="RsScope_rngPCIeTLPSnoop", "Read Callback"="rsscope_FormatSearchNameInt32_ReadCallback.vi", "Write Callback"="rsscope_FormatSearchNameInt32_WriteCallback.vi", "Supported Models"="RTO|RTP", "Instrument Options"="K72", "Flags"=0, "Help"="Sets the snoop state to be searched for in the transaction layer type.\n\nAvailable Repeated Capabilities:\nNone\n\nRemote-control command(s):\nSEARch:TRIGger:PCIE:TLP:SNOO"}, {"Level"=5, "Class Only"=FALSE, "Identifier"="RSSCOPE_ATTR_PCIE_SEARCH_TLP_REQUESTER_ID", "Descriptive Name"="PCIe Search TLP Requester ID", "Data Type"=2, "Command"="SEAR:TRIG:PCIE:TLP:REID", "Access"=2, "Range Table"="", "Read Callback"="rsscope_FormatSearchNameString_ReadCallback.vi", "Write Callback"="rsscope_FormatSearchNameString_WriteCallback.vi", "Supported Models"="RTO|RTP", "Instrument Options"="K72", "Flags"=0, "Help"="Sets the requester ID to be searched for in the transaction layer type.\n\nAvailable Repeated Capabilities:\nNone\n\nRemote-control command(s):\nSEARch:TRIGger:PCIE:TLP:REID"}, {"Level"=5, "Class Only"=FALSE, "Identifier"="RSSCOPE_ATTR_PCIE_SEARCH_TLP_DEVICE_ID", "Descriptive Name"="PCIe Search TLP Device ID", "Data Type"=2, "Command"="SEAR:TRIG:PCIE:TLP:DEID", "Access"=2, "Range Table"="", "Read Callback"="rsscope_FormatSearchNameString_ReadCallback.vi", "Write Callback"="rsscope_FormatSearchNameString_WriteCallback.vi", "Supported Models"="RTO|RTP", "Instrument Options"="K72", "Flags"=0, "Help"="Sets the device ID to be searched for in the transaction layer type.\n\nAvailable Repeated Capabilities:\nNone\n\nRemote-control command(s):\nSEARch:TRIGger:PCIE:TLP:DEID"}, {"Level"=5, "Class Only"=FALSE, "Identifier"="RSSCOPE_ATTR_PCIE_SEARCH_TLP_READ_WRITE", "Descriptive Name"="PCIe Search TLP Read Write", "Data Type"=0, "Command"="SEAR:TRIG:PCIE:TLP:MERW", "Access"=2, "Range Table"="RsScope_rngPCIeTLPReadWrite", "Read Callback"="rsscope_FormatSearchNameInt32_ReadCallback.vi", "Write Callback"="rsscope_FormatSearchNameInt32_WriteCallback.vi", "Supported Models"="RTO|RTP", "Instrument Options"="K72", "Flags"=0, "Help"="Sets the read/ write type to be searched for in the transaction layer type.\n\nAvailable Repeated Capabilities:\nNone\n\nRemote-control command(s):\nSEARch:TRIGger:PCIE:TLP:MERW"}, {"Level"=5, "Class Only"=FALSE, "Identifier"="RSSCOPE_ATTR_PCIE_SEARCH_TLP_ADDRESS_TYPE", "Descriptive Name"="PCIe Search TLP Address Type", "Data Type"=0, "Command"="SEAR:TRIG:PCIE:TLP:ADRT", "Access"=2, "Range Table"="RsScope_rngPCIeTLPAddressType", "Read Callback"="rsscope_FormatSearchNameInt32_ReadCallback.vi", "Write Callback"="rsscope_FormatSearchNameInt32_WriteCallback.vi", "Supported Models"="RTO|RTP", "Instrument Options"="K72", "Flags"=0, "Help"="Sets the address type to be searched for in the transaction layer type.\n\nAvailable Repeated Capabilities:\nNone\n\nRemote-control command(s):\nSEARch:TRIGger:PCIE:TLP:ADRT"}, {"Level"=5, "Class Only"=FALSE, "Identifier"="RSSCOPE_ATTR_PCIE_SEARCH_TLP_TYPE", "Descriptive Name"="PCIe Search TLP Type", "Data Type"=0, "Command"="SEAR:TRIG:PCIE:TLP:CFGT", "Access"=2, "Range Table"="RsScope_rngPCIeTLPType", "Read Callback"="rsscope_FormatSearchNameInt32_ReadCallback.vi", "Write Callback"="rsscope_FormatSearchNameInt32_WriteCallback.vi", "Supported Models"="RTO|RTP", "Instrument Options"="K72", "Flags"=0, "Help"="Sets the configuration type to be searched for in the transaction layer type.\n\nAvailable Repeated Capabilities:\nNone\n\nRemote-control command(s):\nSEARch:TRIGger:PCIE:TLP:CFGT"}, {"Level"=5, "Class Only"=FALSE, "Identifier"="RSSCOPE_ATTR_PCIE_SEARCH_TLP_ROUTING", "Descriptive Name"="PCIe Search TLP Routing", "Data Type"=0, "Command"="SEAR:TRIG:PCIE:TLP:MSGR", "Access"=2, "Range Table"="RsScope_rngPCIeTLPRouting", "Read Callback"="rsscope_FormatSearchNameInt32_ReadCallback.vi", "Write Callback"="rsscope_FormatSearchNameInt32_WriteCallback.vi", "Supported Models"="RTO|RTP", "Instrument Options"="K72", "Flags"=0, "Help"="Sets the message routing type to be searched for in the transaction layer type.\n\nAvailable Repeated Capabilities:\nNone\n\nRemote-control command(s):\nSEARch:TRIGger:PCIE:TLP:MSGR"}, {"Level"=5, "Class Only"=FALSE, "Identifier"="RSSCOPE_ATTR_PCIE_SEARCH_TLP_MESSAGE_CODE", "Descriptive Name"="PCIe Search TLP Message Code", "Data Type"=2, "Command"="SEAR:TRIG:PCIE:TLP:MSGC", "Access"=2, "Range Table"="", "Read Callback"="rsscope_FormatSearchNameString_ReadCallback.vi", "Write Callback"="rsscope_FormatSearchNameString_WriteCallback.vi", "Supported Models"="RTO|RTP", "Instrument Options"="K72", "Flags"=0, "Help"="Sets the message code to be searched for in the transaction layer type.\n\nAvailable Repeated Capabilities:\nNone\n\nRemote-control command(s):\nSEARch:TRIGger:PCIE:TLP:MSGC"}, {"Level"=5, "Class Only"=FALSE, "Identifier"="RSSCOPE_ATTR_PCIE_SEARCH_TLP_STATUS", "Descriptive Name"="PCIe Search TLP Status", "Data Type"=0, "Command"="SEAR:TRIG:PCIE:TLP:CPLS", "Access"=2, "Range Table"="RsScope_rngPCIeTLPStatus", "Read Callback"="rsscope_FormatSearchNameInt32_ReadCallback.vi", "Write Callback"="rsscope_FormatSearchNameInt32_WriteCallback.vi", "Supported Models"="RTO|RTP", "Instrument Options"="K72", "Flags"=0, "Help"="Sets the completion status to be searched for in the transaction layer type.\n\nAvailable Repeated Capabilities:\nNone\n\nRemote-control command(s):\nSEARch:TRIGger:PCIE:TLP:CPLS"}, {"Level"=5, "Class Only"=FALSE, "Identifier"="RSSCOPE_ATTR_PCIE_SEARCH_TLP_COMPLETER_ID", "Descriptive Name"="PCIe Search TLP Completer ID", "Data Type"=2, "Command"="SEAR:TRIG:PCIE:TLP:CPID", "Access"=2, "Range Table"="", "Read Callback"="rsscope_FormatSearchNameString_ReadCallback.vi", "Write Callback"="rsscope_FormatSearchNameString_WriteCallback.vi", 
